vi "pHCheck.vi"() -> ()   [LabVIEW 2016]
panel:
  out "Even/Odd":string
  in  "Numeric":dbl
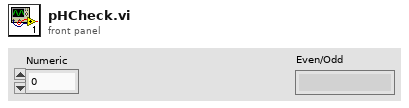
[diagram p1: front panel]
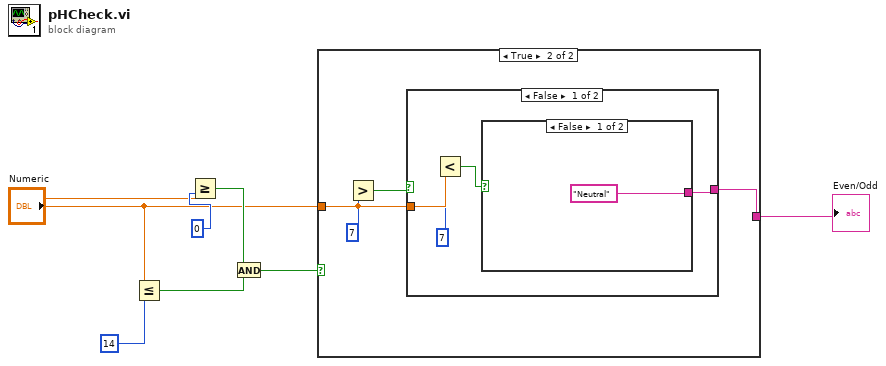
[diagram p0: block diagram]
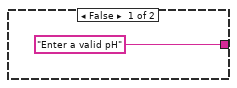
[diagram p2: hidden frame]
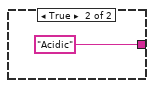
[diagram p3: hidden frame]
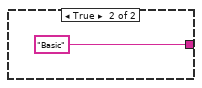
[diagram p4: hidden frame]
diagram:
  n1 = Less Or Equal?(x="Numeric", y=14) -> (x <= y?=w4:bool)
  n2 = Greater Or Equal?(x="Numeric", y=0) -> (x >= y?=w3:bool)
  n3 = And(x=w3, y=w4) -> (x .and. y?=w2:bool)
  n4 = case shown="True" w2 {
    tunnel: ["Enter a valid pH" w10] -> w7
    tunnel: "Numeric" -> [_ w9]
    frame False {
    }
    frame True {
      n5 = Greater?(x=w9, y=7) -> (0:w11:bool)
      n6 = case shown="False" w11 {
        tunnel: [w13 "Basic"] -> w10
        tunnel: w9 -> [w15 _]
        frame False {
          n7 = Less?(x=w15, y=7) -> (x < y?=w16:bool)
          n8 = case shown="False" w16 {
            tunnel: ["Neutral" "Acidic"] -> w13
            frame False {
            }
            frame True {
            }
          }
        }
        frame True {
        }
      }
    }
  }
  "Even/Odd" <- w7
